vi "testFlattenTemperatureAbsToXML.vi"() -> ()   [LabVIEW 2012, in "UnitsAndXML.lvlib"]
uses:
  <userlib>/Common/UnitsAndXML/UnitsAndXML.lvlib
  <userlib>/Common/UnitsAndXML/FlattenItemWithUnitToXML/FlattenTemperatureAbsToXML/TemperatureAbsUnit.ctl
  <userlib>/Common/UnitsAndXML/FlattenItemWithUnitToXML/FlattenTemperatureAbsToXML/typeMethods/flattenTemperatureAbsToXML_Array.vi
  <userlib>/Common/UnitsAndXML/FlattenItemWithUnitToXML/FlattenTemperatureAbsToXML/typeMethods/flattenTemperatureAbsToXML_Scalar.vi
panel:
  out "error out":errorcluster
  in  "temperatureAbsUnitInXML":T1
  out "xmlStringArray":string
  out "xmlStringScalar":string
  in  "temperatureAbs":dbl[unit][](array[numeric])=[288.15, 303.15, 318.15, 333.15]
  in  "temperatureAbs":dbl[unit]=288.15
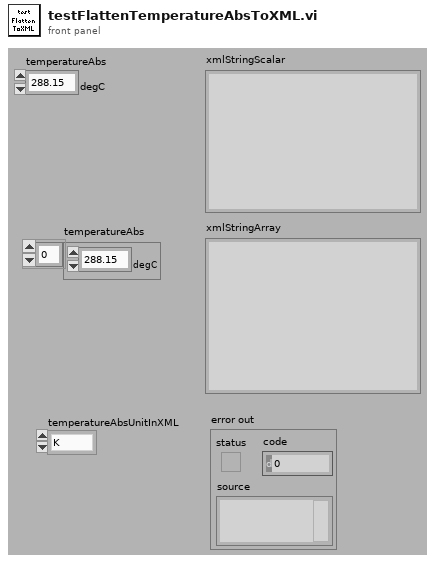
[diagram p1: front panel]
types:
  T1 = typedef "UnitsAndXML.lvlib/TemperatureAbsUnit.ctl" = enum16{"K", "degC", "degF"}
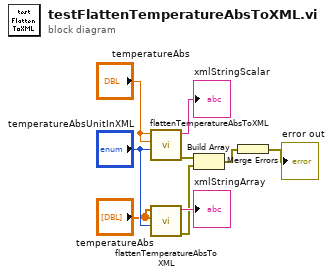
[diagram p0: block diagram]
diagram:
  n1 = call-poly <userlib>:"flattenTemperatureAbsToXML.vi"("temperatureAbsUnitInXML"="temperatureAbsUnitInXML", "temperatureAbsAgain"="temperatureAbs", "temperatureAbs"="temperatureAbs") -> ("error out"=w6:errorcluster, "xmlString"=→"xmlStringScalar":string)  [unwired: 7 in]
  n2 = call-poly <userlib>:"flattenTemperatureAbsToXML.vi"("temperatureAbsUnitInXML"="temperatureAbsUnitInXML", "temperatureAbsAgain"="temperatureAbs", "temperatureAbs"="temperatureAbs") -> ("error out"=w1:errorcluster, "xmlString"=→"xmlStringArray":string)  [unwired: 7 in]
  n3 = Build Array(w6, w1) -> (w7:errorcluster[])
  n4 = Merge Errors(w7) -> (→"error out":errorcluster)
